vi "PDHydra - PWM NODC Test_v2.vi"(8 "error in (no error) 2":errorcluster, 10 "HMP4040 VISA":refnum<visa-resource-name>, 11 "Control Board VISA":refnum<visa-resource-name>="ControlBoard") -> (0 "error out":errorcluster, 2 "Message OUT":string, 3 "Result (bool)":bool)   [LabVIEW 2022 SP3]
uses:
  Serial Board Com/Board Select.ctl
  HMP4000 Communication/HMP4040_ChannelControlAutomatic.ctl
  <vilib>/DAQmx/read.llb/DAQmx Read (Analog 1D Wfm NChan NSamp).vi
  <vilib>/DAQmx/miscellaneous.llb/DAQmx Fill In Error Info.vi
panel:
  in  "Board Selector":T1
  out "Duty Cycle VISA Write":string[](array[string])
  out "ControlBoard OUT":refnum<visa-resource-name>
  in  "Message IN":string=" "
  out "Analysis Leg":i32
  out "Waveforms":T2
  out "Active Leg":i32
  out "Result (color)":u32(colorbox)
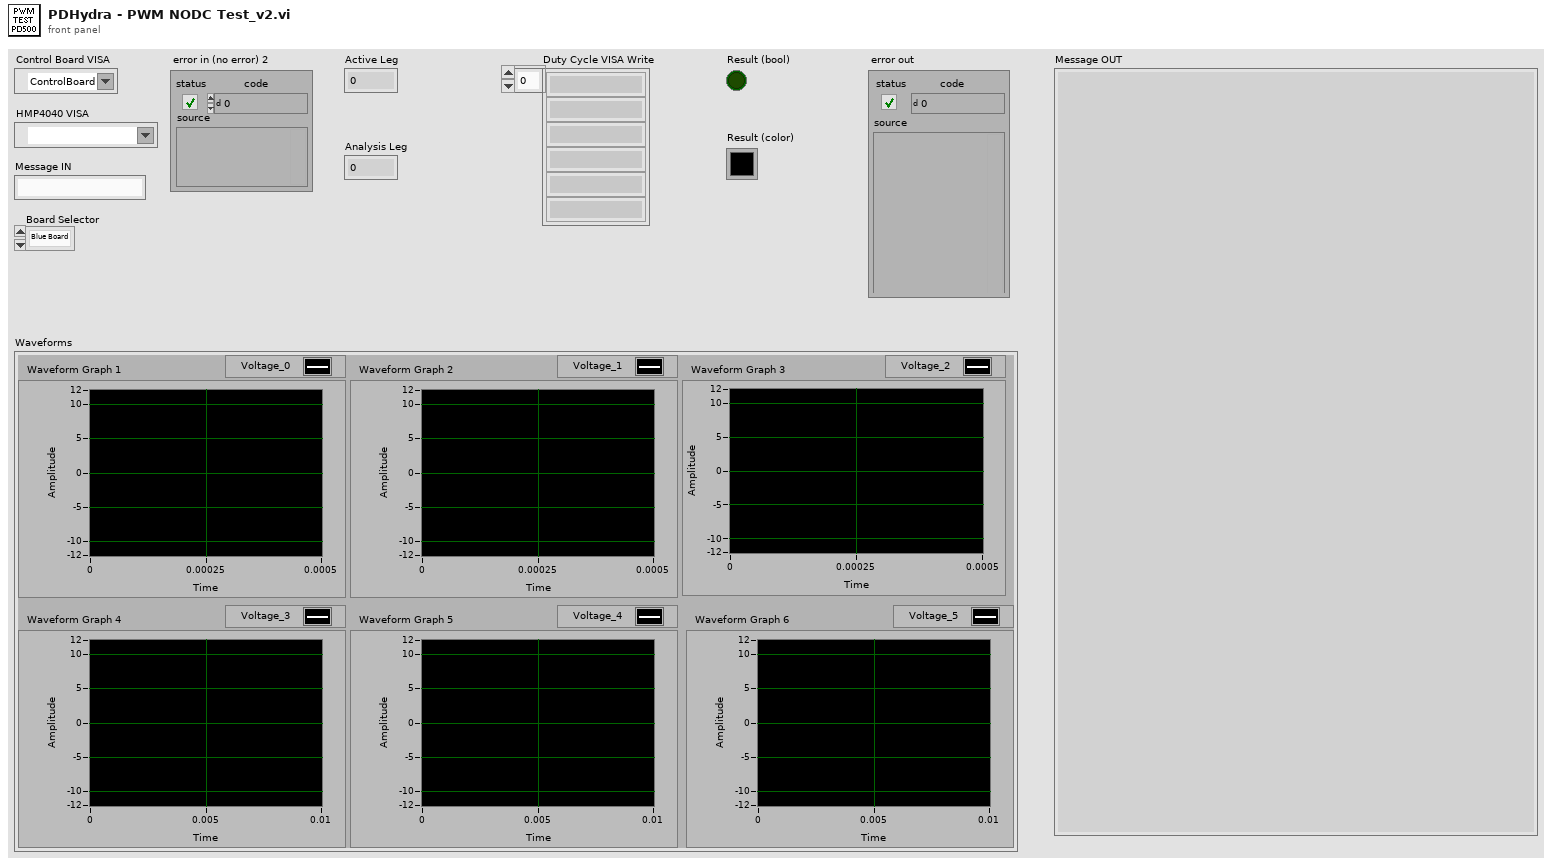
[diagram p1: front panel]
types:
  T1 = typedef "Board Select.ctl" = enum16{"Blue Board", "Green Board"}
  T2 = cluster{"Waveform Graph 1":waveform(dbl), "Waveform Graph 2":waveform(dbl), "Waveform Graph 3":waveform(dbl), "Waveform Graph 4":waveform(dbl), "Waveform Graph 5":waveform(dbl), "Waveform Graph 6":waveform(dbl)}
  T3 = typedef "HMP4040_ChannelControlAutomatic.ctl" = enum16{"Off", "Control Power", "HMP2020 Control + DC32V", "HMP2020 Control + DC8V", "HMP4040 Control + DC32V", "HMP4040 Control +DC8V", "HMP4040 Ch2 24V 4A"}
  T4 = cluster{"data[0]":waveform(dbl), "data[1]":waveform(dbl), "data[2]":waveform(dbl), "data[3]":waveform(dbl), "data[4]":waveform(dbl), "data[5]":waveform(dbl)}
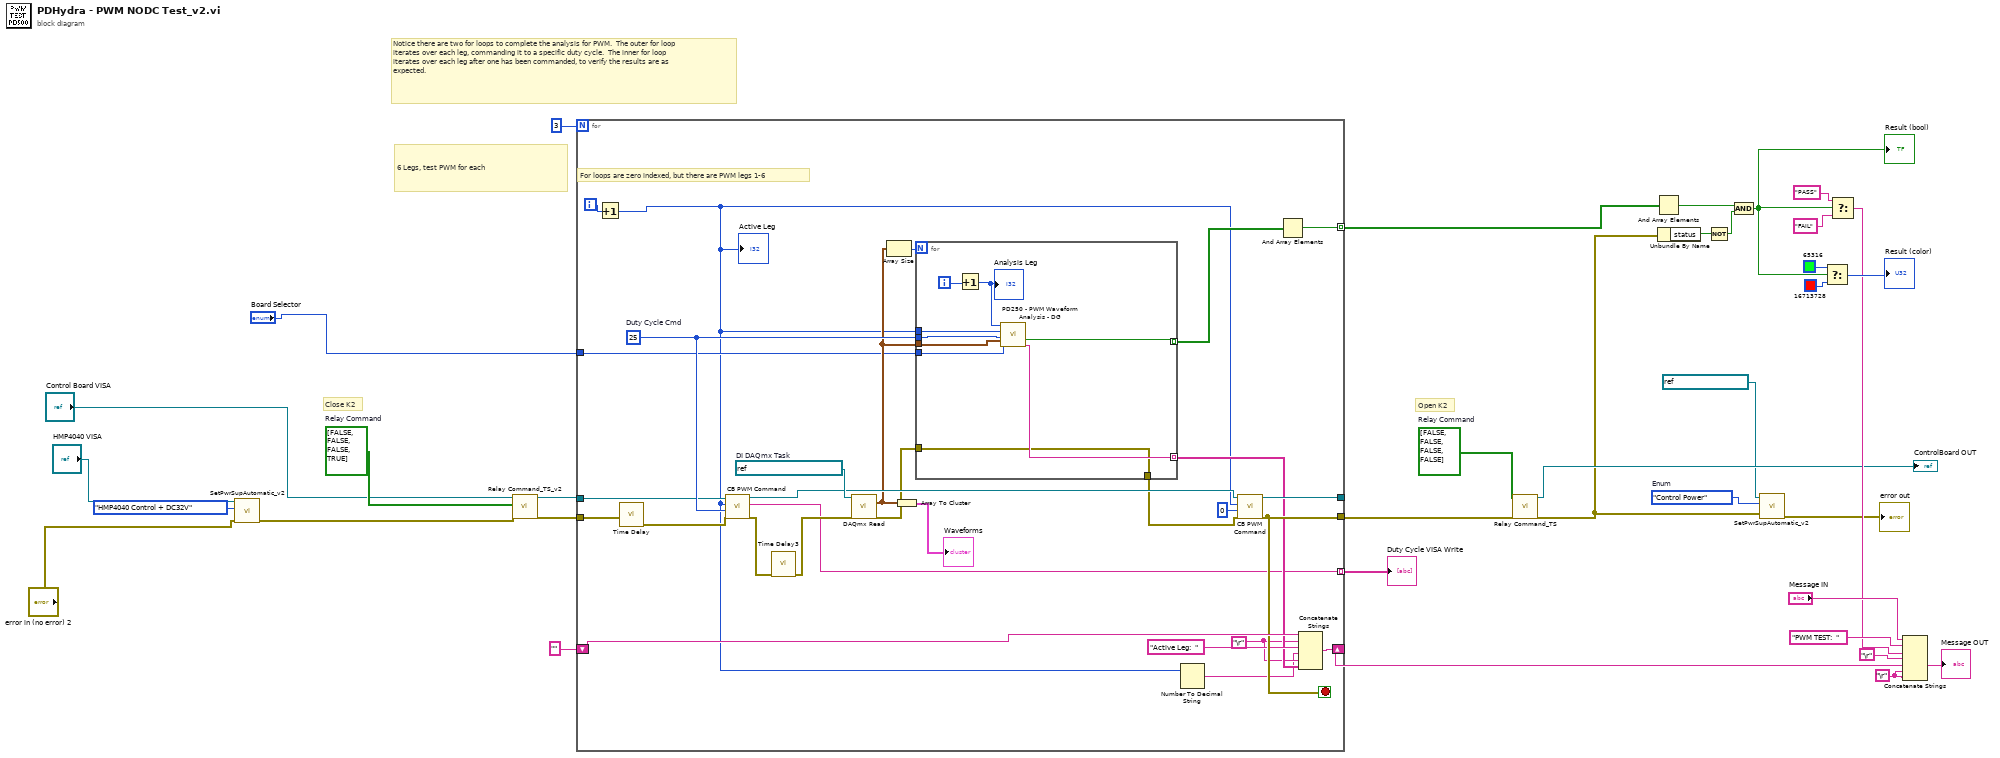
[diagram p0: block diagram]
diagram:
  w4 = HMP4040_ChannelControlAutomatic."Control Power"  # Enum
  w12 = bool[] [FALSE, FALSE, FALSE, TRUE]  # Relay Command
  w5 = bool[] [FALSE, FALSE, FALSE, FALSE]  # Relay Command
  w25 = "\r"
  # "Close K2"
  # "Open K2"
  # "Notice there are two for loops to complete the analysis for PWM.  The outer for loop iterates over each leg, commanding it to a specific duty cycle.  The inner for loop iterates over each leg after one has been commanded, to verify the results are as expected."
  # "6 Legs, test PWM for each"
  n1 = call "SetPwrSupAutomatic_v2.vi"("error in (no error)"="error in (no error) 2", "Enum"=HMP4040_ChannelControlAutomatic."HMP4040 Control + DC32V", "HMP VISA"="HMP4040 VISA") -> ("error out"=w10:errorcluster)  [unwired: 7 in, 1 out]
  n2 = call "Relay Command_TS_v2.vi"("error in (no error)"=w10, "Relay Command"=w12, "Control Board VISA"="Control Board VISA") -> ("error out"=w14:errorcluster, "VISA Refnum out"=w15:refnum<visa-resource-name>)  [unwired: 7 in]
  n3 = for {
    N: 3 -> [_]
    tunnel: [w64] -> w36 mode=indexing
    shift-right: [w62] -> w23
    shift-left: "" -> [w61]
    tunnel: [w57] -> w17
    tunnel: [w52] -> _
    tunnel: w14 -> [w42]
    tunnel: w15 -> [w47]
    tunnel: [w44] -> w13 mode=indexing
    tunnel: "Board Selector" -> [w43]
    i -> [w37]
    stop <- w57 stop-if-true
    w49 = "\r"
    w58 = 25  # Duty Cycle Cmd
    w63 = refnum<k21> "FTS2_PWMInput_DG"  # DI DAQmx Task
    # "For loops are zero indexed, but there are PWM legs 1-6"
    n4 = Increment(x=w37) -> (x+1=w38:i32)
    "Active Leg" <- w38
    n5 = call "Time Delay"("error in (no error)"=w42) -> ("error out"=w41:errorcluster)  [unwired: 10 in]
    n6 = call "CB PWM Command.vi"("error in (no error)"=w41, "Duty Cycle"=w58, "Leg"=w38, "VISA Refnum in"=w47) -> ("error out"=w46:errorcluster, "read buffer"=w44:string, "VISA Refnum out"=w59:refnum<visa-resource-name>)  [unwired: 5 in]
    n7 = call "Time Delay3"("error in (no error)"=w46) -> ("error out"=w45:errorcluster)  [unwired: 10 in]
    n8 = call-poly <vilib>:"DAQmx Read.vi"("task/channels in"=w63, "error in"=w45) -> ("data"=w53:waveform(dbl)[], "error out"=w39:errorcluster)  [unwired: 11 in, 1 out]
    n9 = Array Size(array=w53) -> (size(s)=w54:i32)
    n10 = Array To Cluster(array=w53) -> (cluster=→"Waveforms":T4)
    n11 = for {
      N: w54 -> [_]
      tunnel: w58 -> [w73]
      tunnel: w53 -> [w72]
      tunnel: w38 -> [w71]
      tunnel: [w70] -> w55 mode=indexing
      tunnel: [w69] -> w50 mode=indexing
      tunnel: w43 -> [w68]
      tunnel: [w67] -> w40
      tunnel: w39 -> [w67]
      i -> [w66]
      n12 = Increment(x=w66) -> (x+1=w65:i32)
      "Analysis Leg" <- w65
      n13 = call "PD250 - PWM Waveform Analysis - DG.vi"("Analysis Leg"=w65, "Active Leg"=w71, "Duty Cycle"=w73, "Waveform"=w72, "Board Selector"=w68) -> ("Result (Boolean)"=w70:bool, "Message"=w69:string)  [unwired: 9 in]
    }
    n14 = Number To Decimal String(number=w38) -> (decimal integer string=w48:string)  [unwired: 1 in]
    n15 = call "CB PWM Command.vi"("error in (no error)"=w40, "Duty Cycle"=0, "Leg"=w38, "VISA Refnum in"=w59) -> ("error out"=w57:errorcluster, "VISA Refnum out"=w52:refnum<visa-resource-name>)  [unwired: 5 in, 1 out]
    n16 = And Array Elements(Boolean array=w55) -> (logical AND=w64:bool)
    n17 = Concatenate Strings(w61, w49, "Active Leg:  ", w48, w49, w50) -> (w62:string)
  }
  "Duty Cycle VISA Write" <- w13
  n18 = call "Relay Command_TS.vi"("error in (no error)"=w17, "Relay Command"=w5) -> ("error out"=w8:errorcluster, "VISA Refnum out"=→"ControlBoard OUT":refnum<visa-resource-name>)  [unwired: 8 in]
  n19 = And Array Elements(Boolean array=w36) -> (logical AND=w26:bool)
  n20 = Unbundle By Name(w8) -> ("status"=w29:bool)
  n21 = Not(x=w29) -> (.not. x?=w28:bool)
  n22 = And(x=w26, y=w28) -> (x .and. y?=w27:bool)
  "Result (bool)" <- w27
  n23 = call "SetPwrSupAutomatic_v2.vi"("error in (no error)"=w8, "Enum"=w4, "HMP VISA"=refnum<visa-resource-name> "HMP4040_FTS2" ("VISA resource name")) -> ("error out"=→"error out":errorcluster)  [unwired: 7 in, 1 out]
  n24 = Select(t=u32 65316 ("Result (color)"), s=w27, f=u32 16713728 ("Result (color)")) -> (s? t:f=→"Result (color)":u32)
  n25 = Select(t="PASS", s=w27, f="FAIL") -> (s? t:f=w18:string)
  n26 = Concatenate Strings("Message IN", "PWM TEST:  ", w18, "\r", w23, w25, w25) -> (→"Message OUT":string)
